vi "Take Portion of Data (multiple).vi"(8 "error in (no error)":errorcluster, 9 "Method":enum16{"Slider (%)", "X[] min and max"}(ring), 10 "Slider":cluster{dbl, dbl}(slide)={0.0, 0.5348837209302325} caption="Horizontal Slider" scale=0.0..1.0, 11 "Multiple XY-data in":cluster{"X-array":dbl[], "Y-array":dbl[]}[](array[cluster]) {"Y-array" format="%.2p"; "X-array" format="%.2p"}) -> (0 "error out":errorcluster, 3 "Multiple XY-data out":cluster{"X-array":dbl[], "Y-array":dbl[]}[](array[cluster]) {"Y-array" format="%.2p"; "X-array" format="%.2p"})   [LabVIEW 2016, in "xy_utilities.lvlib"]
uses:
  xy_utilities.lvlib
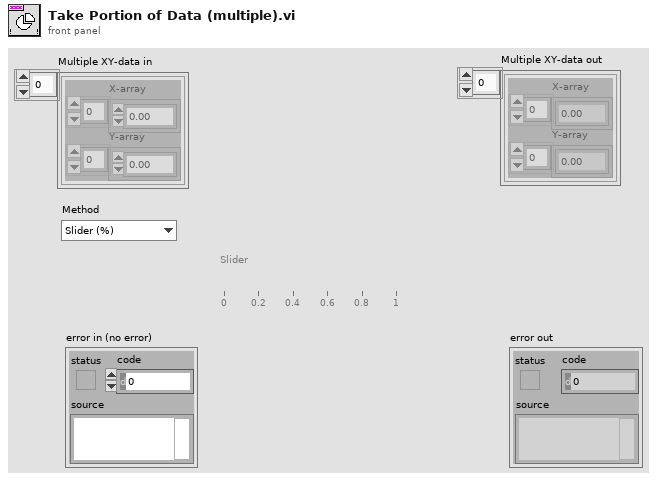
[diagram p1: front panel]
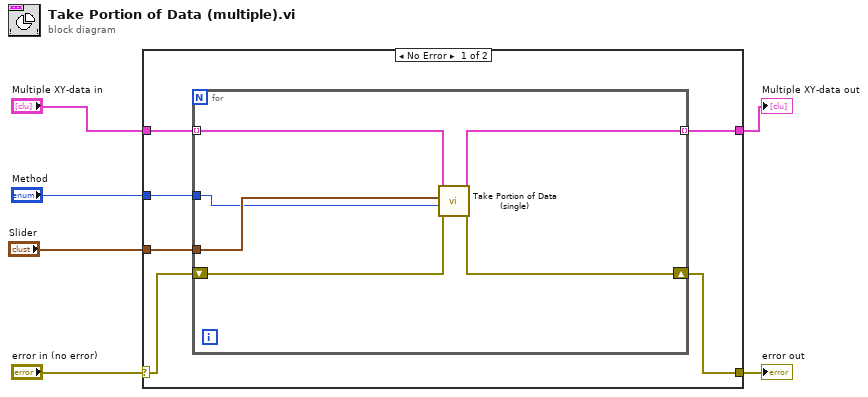
[diagram p0: block diagram]
diagram:
  n1 = case shown="No Error" "error in (no error)" {
    selector: "error in (no error)" -> [w8 w20]
    tunnel: [w7 w20] -> w5
    tunnel: "Multiple XY-data in" -> [w12 w19]
    tunnel: [w9 w19] -> w3
    tunnel: "Method" -> [w10 _]
    tunnel: "Slider" -> [w11 _]
    frame No Error {
      n2 = for {
        tunnel: w12 -> [w14] mode=indexing
        tunnel: w11 -> [w18]
        tunnel: w10 -> [w17]
        tunnel: [w13] -> w9 mode=indexing
        shift-right: [w15] -> w7
        shift-left: w8 -> [w16]
        n3 = call "Take Portion of Data (single).vi"("error in (no error)"=w16, "Method"=w17, "Slider"=w18, "XY-data in"=w14) -> ("error out"=w15:errorcluster, "XY-data out"=w13:cluster{"X-array":dbl[], "Y-array":dbl[]})  [unwired: 6 in]
      }
    }
    frame Error {
    }
  }
  "error out" <- w5
  "Multiple XY-data out" <- w3
